vi "Process_Application.vi"(5 "Splash StatusRef":refnum<vi>, 7 "Splash VI Ref":refnum<vi>, 9 "Simulation?":bool, 10 "LaunchState Ev":refnum<user-event>) -> ()   [LabVIEW 2019, in "Application.lvclass"]
doc: "Developed by Kevin Thompson\nkevin@thompsonengineering.net\n\nCopyright 2018\nThompson Engineering, LLC"
uses:
  Application.lvclass
  <vilib>/TELLC/SMQ/Add States to Queue using MultiLine String with vData.vi
  DataTypes/Process - AppData--cluster.ctl
  Common/DataTypes/TD Async CmdMsg EventData--cluster.ctl
  DataTypes/Public Events--cluster.ctl
  DataTypes/Dependency--cluster.ctl
  DataTypes/Settings--cluster.ctl
  Common/Startup/TD LaunchState--enum.ctl
  Common/Startup/TD LaunchData--cluster.ctl
  Common/ErrorHandler/ErrorHandler.lvclass
  Common/DataTypes/TD GetSet ActionSelect--enum.ctl
  Subsystems/Log_Engine/Log_Engine.lvclass
  Subsystems/DAQ_Engine/DAQ_Engine.lvclass
  Subsystems/Main/Main.lvclass
  Subsystems/Config/Config.lvclass
  DataTypes/Read Data--cluster.ctl
panel:
  in  "localData":cluster{"Msg":string, "vData":variant}
  in  "process sync":refnum<notifier>
  out "Application ReadData":T1
  in  "Exit":bool
  in  "Application in":refnum<class "Application.lvclass">
  # "local data monitoring"
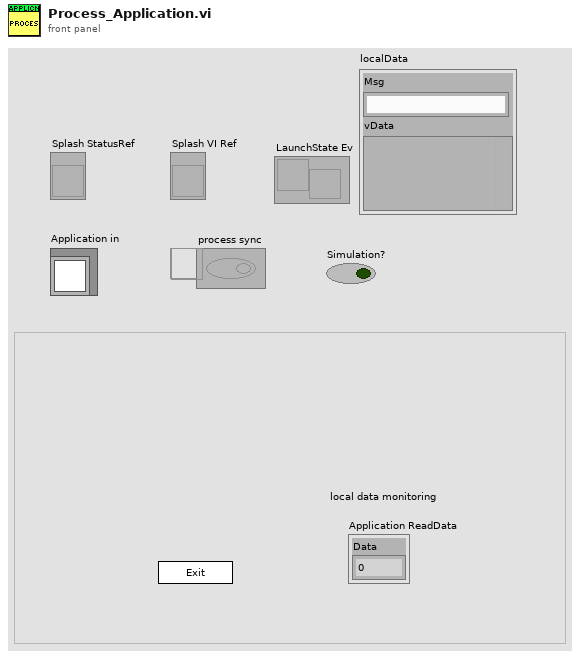
[diagram p1: front panel]
types:
  T1 = typedef "Application.lvclass/Read Data--cluster.ctl" = cluster{"Data":dbl}
  T2 = typedef "TD LaunchData--cluster.ctl" = cluster{"Time Stamp":timestamp, "LaunchState":T3, "Error":errorcluster}
  T3 = typedef "TD LaunchState--enum.ctl" = enum16{"Started", "Stopped"}
  T4 = typedef "Application.lvclass/Process - AppData--cluster.ctl" = cluster{"Core":cluster{"Current VI Reference":refnum<vi>, "Close Panel on Exit?":bool}, "Your Boolean data":bool, "Your string data":string, "SMQ":refnum<queue>, "Initialized?":bool, "Self Reference":refnum<class "Application.lvclass">, "Simulation?":bool, "process sync":refnum<notifier>, "vData":variant, "Public Events":T5, "LaunchState Ev":refnum<user-event>, "RunTimeSystem":bool, "ErrorHandler":refnum<class "ErrorHandler.lvclass">, "Dependency":T6, "StatusMsg Ref":refnum<vi>, "AO IONames":T7, "DO IONames":T8, "UI Labels":T9, "quitting":bool, "DAQEnabled":bool, "Splash StatusRef":refnum<vi>, "Splash VI Ref":refnum<vi>}
  T5 = typedef "Application.lvclass/Public Events--cluster.ctl" = cluster{"Application.AsyncCmd Event":refnum<user-event>, "Application.AsyncMsg Event":refnum<user-event>, "stop process":refnum<user-event>, "Application.ControlStateChg Event":refnum<user-event>, "Application.RadialGraph Event":refnum<user-event>}
  T6 = typedef "Application.lvclass/Dependency--cluster.ctl" = cluster{"Config":refnum<class "Config.lvclass">, "DAQ":refnum<class "DAQ.lvclass">, "Sequencer":refnum<class "Sequencer.lvclass">, "LogEngine":refnum<class "LogEngine.lvclass">, "ErrorHandler":refnum<class "ErrorHandler.lvclass">, "DataQueues":refnum<class "DataQueues.lvclass">, "Motion":refnum<class "Motion.lvclass">, "PID_Ctlr":refnum<class "PID_Ctlr.lvclass">, "Welder":refnum<class "Welder.lvclass">}
  T7 = typedef "AO IONames--cluster.ctl" = cluster{"Weld Current":string, "Turntable Speed":string, "Turntable Jog":string}
  T8 = typedef "DO IONames--cluster.ctl" = cluster{"Arc Enable Relay":string, "AVC Lockout Relay":string, "Turntable Enable Relay":string, "Turntable Jog Switch":string}
  T9 = typedef "UI Controls-Indicators Labels--cluster.ctl" = cluster{"SeqRunning":string, "Process Complete":string, "AVC Lockout":string, "Step Comment":string, "StepCntDn":string, "SeqList":string, "Current SP":string, "VspOffset":string, "WeldCurrentWfmChart":string, "Turntable En (Anlg)":string}
  T10 = typedef "Application.lvclass/Process - AppData--cluster.ctl" = cluster{"Core":cluster{"Current VI Reference":refnum<vi>, "Close Panel on Exit?":bool}, "Your Boolean data":bool, "Your string data":string, "SMQ":refnum<queue>, "Initialized?":bool, "Self Reference":refnum<class "Application.lvclass">, "Simulation?":bool, "process sync":refnum<notifier>, "vData":variant, "Settings":T11, "Dependency":T12, "Public Events":T13, "Splash StatusRef":refnum<vi>, "Splash VI Ref":refnum<vi>, "LaunchState Ev":refnum<user-event>, "ErrorHandler":refnum<class "ErrorHandler.lvclass">, "RunTimeSystem?":bool, "StatusMsg Ref":refnum<vi>}
  T11 = typedef "Application.lvclass/Settings--cluster.ctl" = cluster{"Simulation":bool}
  T12 = typedef "Application.lvclass/Dependency--cluster.ctl" = cluster{"Config":refnum<class "Config.lvclass">, "Main":refnum<class "Main.lvclass">, "ErrorHandler":refnum<class "ErrorHandler.lvclass">, "DAQ_Engine":refnum<class "DAQ_Engine.lvclass">, "Log_Engine":refnum<class "Log_Engine.lvclass">}
  T13 = typedef "Application.lvclass/Public Events--cluster.ctl" = cluster{"Application.AsyncCmd Event":refnum<user-event>, "Application.AsyncMsg Event":refnum<user-event>, "stop process":refnum<user-event>}
  T14 = typedef "TELLC_Temp01.lvclass/Settings--cluster.ctl" = cluster{"Simulation":bool}
  T15 = enum32{"invalid app kind", "Development System", "Run Time System", "Student Edition", "Embedded LabVIEW", "Evaluation", "Custom"}
  T16 = typedef "TD GetSet ActionSelect--enum.ctl" = enum16{"Init", "Get", "Set"}
  T17 = enum32{"Invalid", "Standard", "Closed", "Hidden", "Minimized", "Maximized"}
  T18 = enum32{"Invalid", "Default", "Floating", "Floating/Auto-Hide", "Modal"}
  T19 = typedef "Application.lvclass/AsynCmd_Application--enum.ctl" = enum16{"Application.DoSomething"}
  T20 = typedef "Application.lvclass/AsynMsg_Application--enum.ctl" = enum16{"Application.AppClassReference"}
  T21 = cluster{"Current VI Reference":refnum<vi>, "Close Panel on Exit?":bool}
  T22 = typedef "TD Pathnames--cluster.ctl" = cluster{"RunTimeSys?":bool, "AppFolder":path, "ExecutablePath":path, "ConfigFolder":path, "DataLogFolder":path, "SystemLogFolder":path, "SeqFolder":path, "MainStartupPathname":path, "MainUIPathname":path, "SystemEventsFile":path, "SeqEventsFile":path, "Config SettingsFile":path, "DAQ IOConfigFile":path, "SystemSimulation":bool}
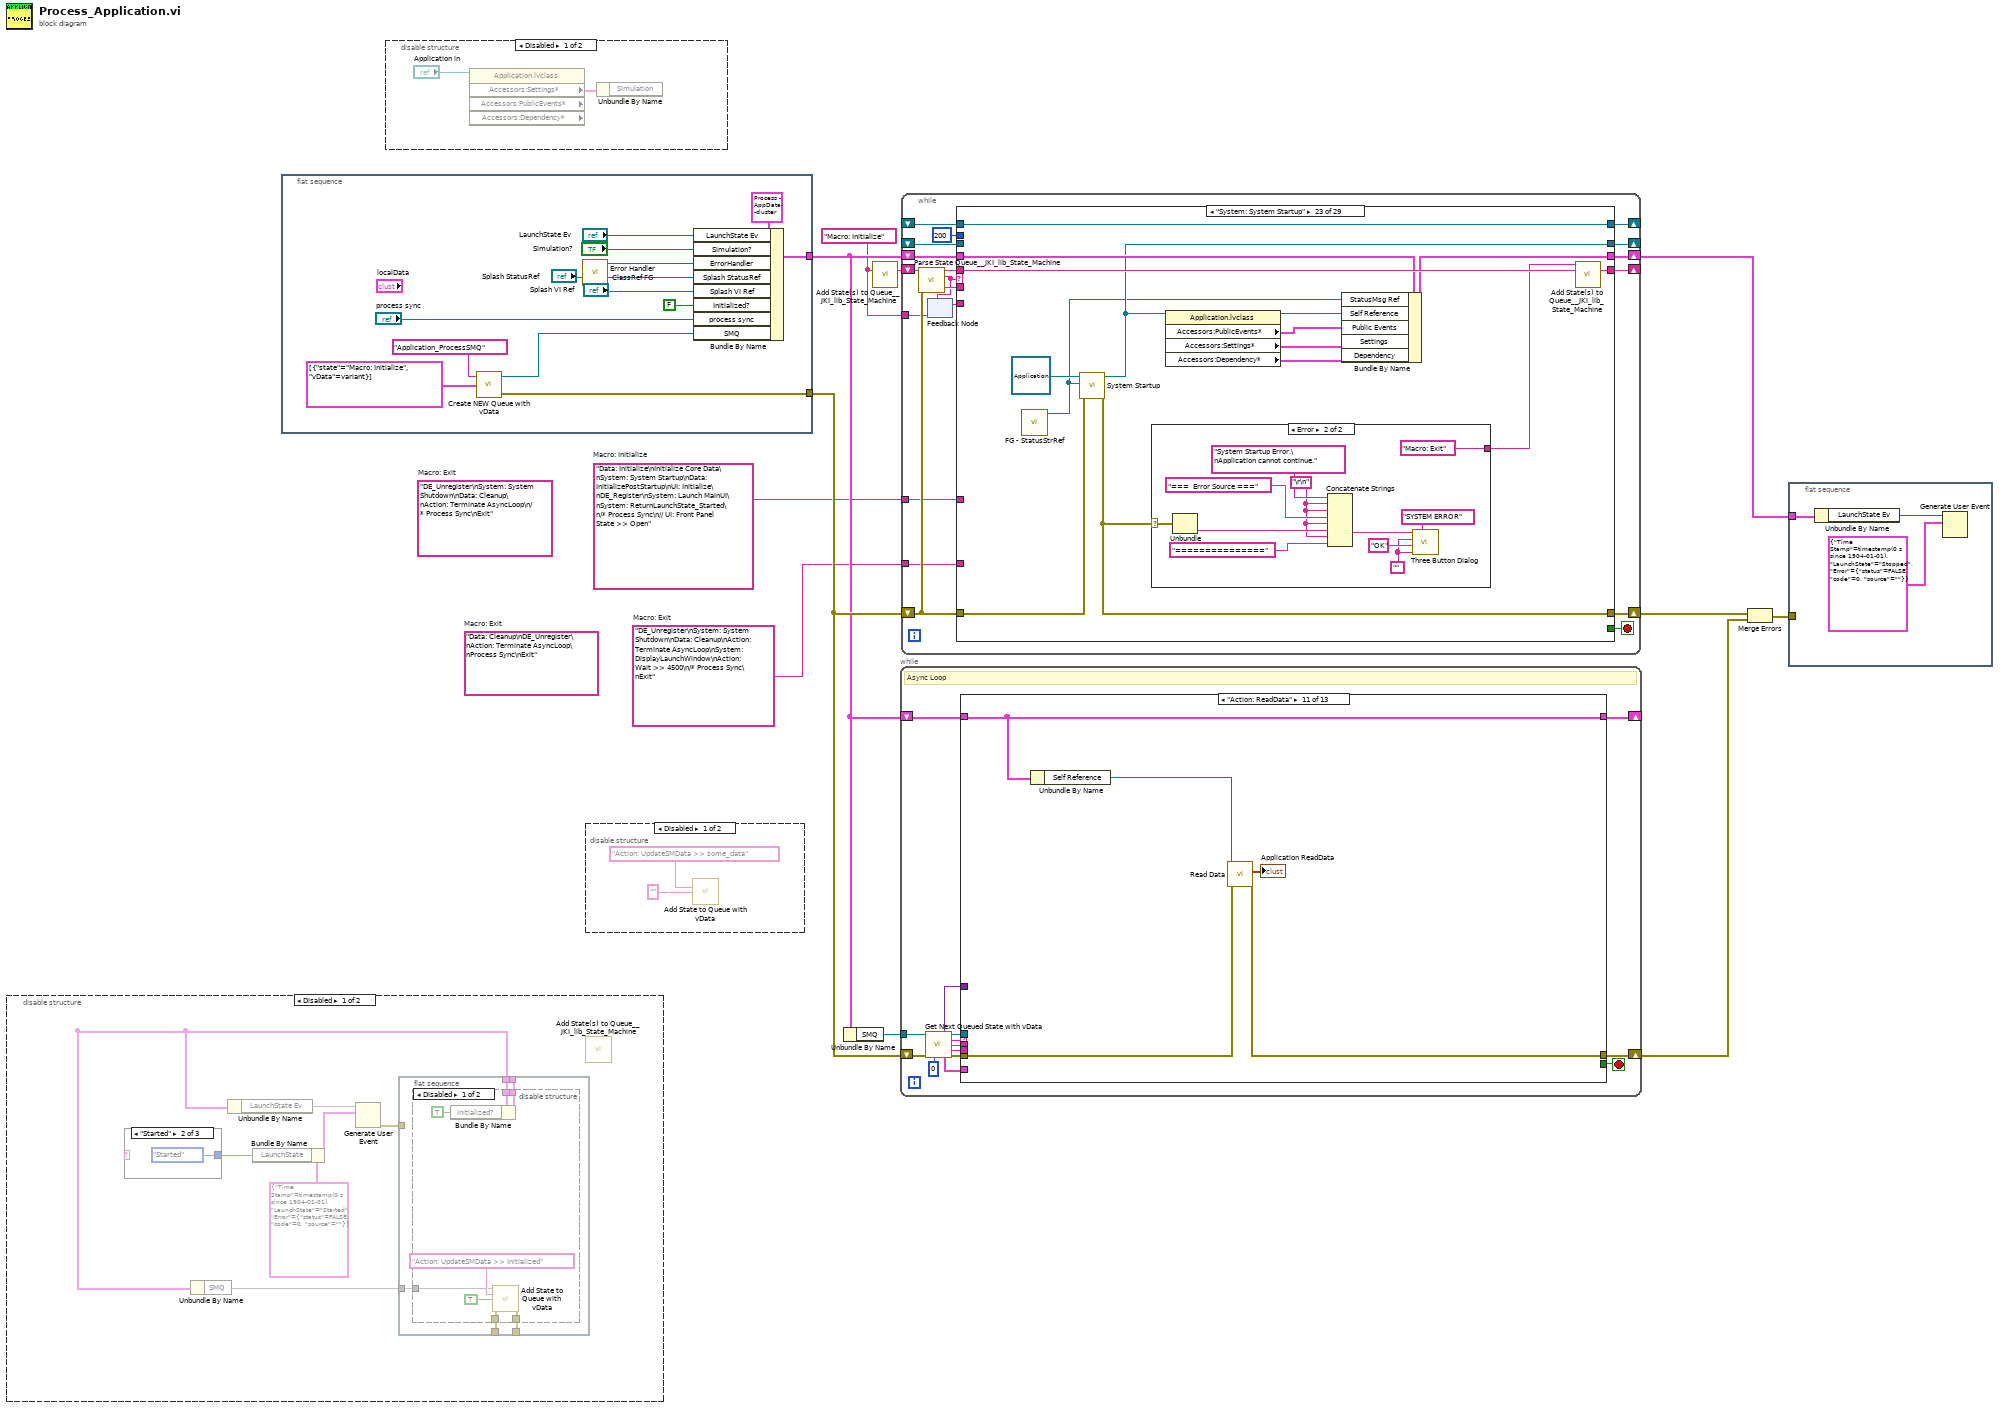
[diagram p0: block diagram]
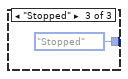
[diagram p4: hidden frame]
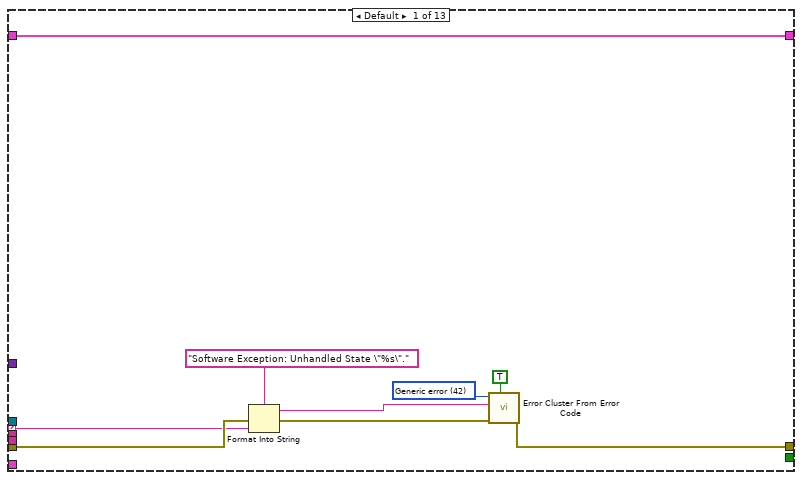
[diagram p8: hidden frame]
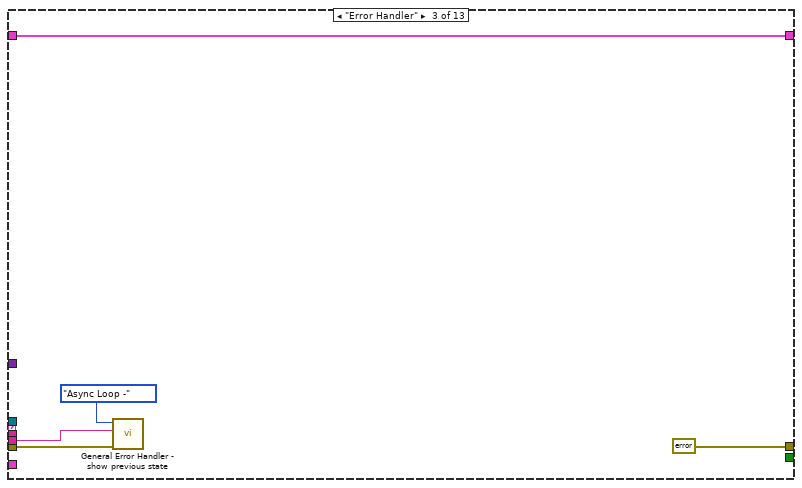
[diagram p10: hidden frame]
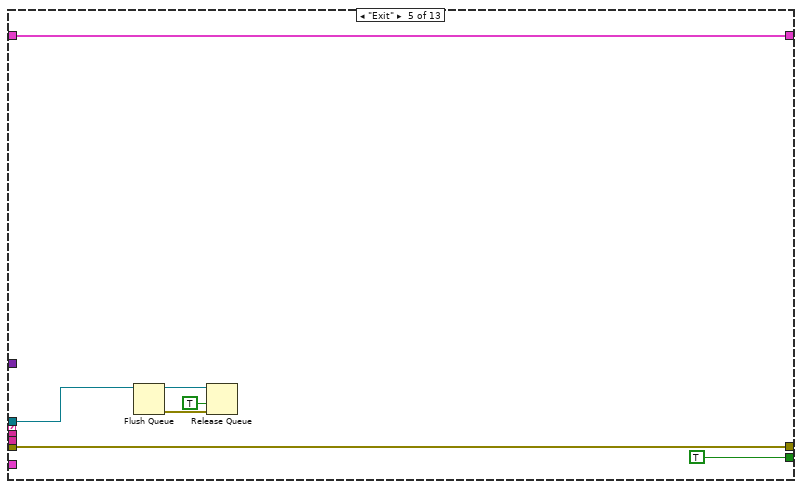
[diagram p12: hidden frame]
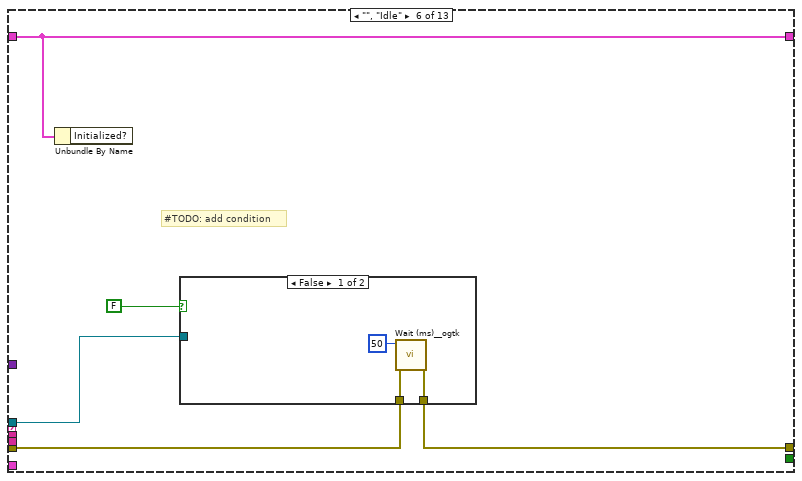
[diagram p13: hidden frame]
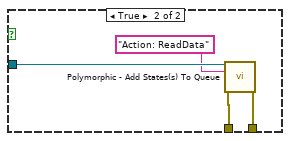
[diagram p14: hidden frame]
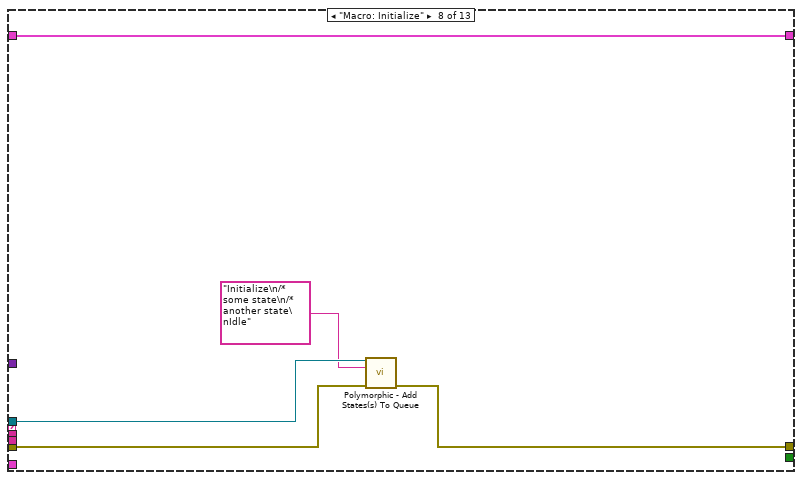
[diagram p16: hidden frame]
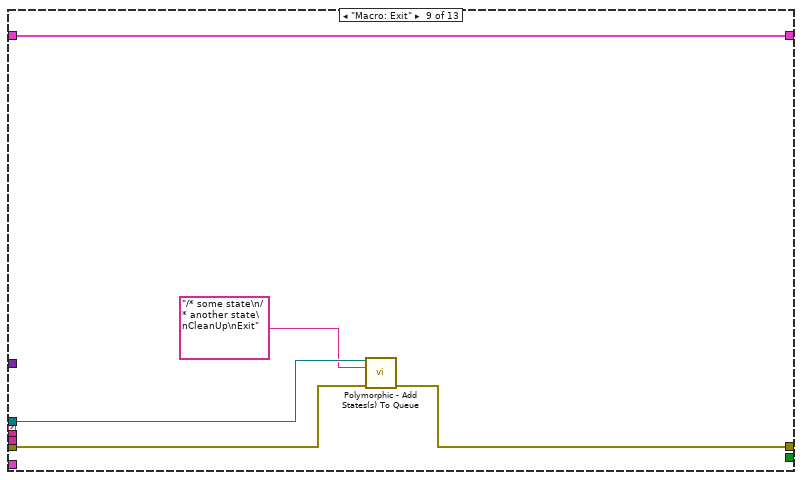
[diagram p17: hidden frame]
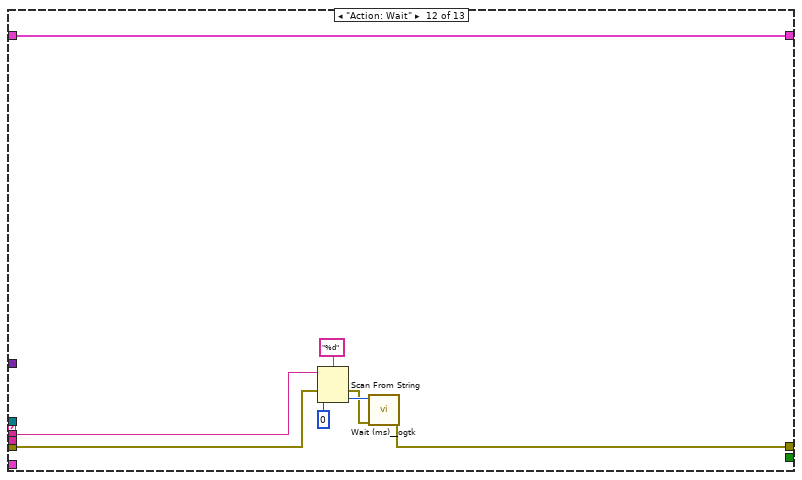
[diagram p19: hidden frame]
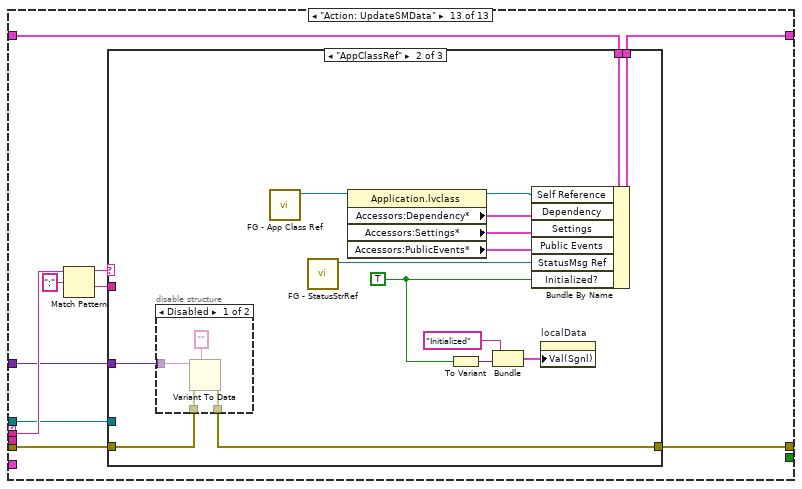
[diagram p20: hidden frame]
diagram:
  w3 = "DE_Unregister\nSystem: System Shutdown\nData: Cleanup\nAction: Terminate AsyncLoop\nSystem: DisplayLaunchWindow\nAction: Wait >> 4500\n/* Process Sync\nExit"  # Macro: Exit
  (unwired) "DE_Unregister\nSystem: System Shutdown\nData: Cleanup\nAction: Terminate AsyncLoop\n/* Process Sync\nExit"  # Macro: Exit
  w4 = "Data: Initialize\nInitialize Core Data\nSystem: System Startup\nData: InitializePostStartup\nUI: Initialize\nDE_Register\nSystem: Launch MainUI\nSystem: ReturnLaunchState_Started\n/* Process Sync\n// UI: Front Panel State >> Open"  # Macro: Initialize
  (unwired) "Data: Cleanup\nDE_Unregister\nAction: Terminate AsyncLoop\nProcess Sync\nExit"  # Macro: Exit
  w5 = "Macro: Initialize"
  n1 = disable-structure shown="Disabled" {
    frame Disabled {
      n2 = case shown="\"Started\"" w19 {
        tunnel: [_ TD_LaunchState--enum."Started" ("LaunchState") TD_LaunchState--enum."Stopped" ("LaunchState")] -> w22
        frame Default {
        }
        frame "Started" {
        }
        frame "Stopped" {
        }
      }
      n3 = Unbundle By Name() -> (w13:T4, "LaunchState Ev"=w20)
      n4 = Unbundle By Name(w13) -> ("SMQ"=w12)
      n5 = Bundle By Name(cluster=T2 {"Time Stamp"=timestamp(0 s since 1904-01-01), "LaunchState"=enum."Started", "Error"={"status"=FALSE, "code"=0, "source"=""}} ("LaunchData"), "LaunchState"=w22) -> (w21:T2)
      n6 = Generate User Event(user event=w20, event data cluster=w21) -> (error out=w16:errorcluster)  [unwired: 2 in, 1 out]
      n7 = flat-sequence {
        tunnel: w13 -> [w28]
        tunnel: [w27] -> w17
        tunnel: w16 -> [_]
        tunnel: [w26] -> w15
        tunnel: [w25] -> w14
        tunnel: w12 -> [w24]
        frame #0 {
          n8 = disable-structure shown="Disabled" {
            disable-tunnel: w28 -> [w36 w38]
            disable-tunnel: [w35 w38] -> w27
            disable-tunnel: w26 -> [w31 w37]
            disable-tunnel: [w30 w37] -> w25
            disable-tunnel: w24 -> [w29 _]
            frame Disabled {
              n9 = Bundle By Name(cluster=w36, "Initialized?"=TRUE) -> (w35:cluster{})
              n10 = call <vilib>:"Add State to Queue with vData.vi"("queue in"=w29, "state in"="Action: UpdateSMData >> Initialized", "vData (\"\")"=TRUE, "error in"=w31) -> ("error out"=w30:errorcluster)  [unwired: 8 in, 3 out]
            }
            frame Enabled {
            }
          }
        }
      }
      n11 = call <vilib>:"Add State(s) to Queue__JKI_lib_State_Machine.vi"() -> ("State(s) in (\"\")"=w23:string)  [unwired: 14 in, 1 out]
    }
    frame Enabled {
    }
  }
  n12 = flat-sequence {
    tunnel: [w53] -> w8
    tunnel: [w50] -> w10
    frame #0 {
      n13 = call <vilib>:"Create NEW Queue with vData.vi"("Initial States"=cluster{"state":string, "vData":variant}[] [{"state"="Macro: Initialize", "vData"=variant}], "Name (SMQ)"="Application_ProcessSMQ") -> ("error out"=w50:errorcluster, "queue out"=w52:refnum<queue>)  [unwired: 2 in]
      n14 = call "Error Handler ClassRef FG.vi"() -> ("ErrorHandler out"=w43:refnum<class "ErrorHandler.lvclass">)  [unwired: 10 in, 1 out]
      n15 = Bundle By Name(cluster=T10 {"Core"={"Current VI Reference"=refnum, "Close Panel on Exit?"=FALSE}, "Your Boolean data"=FALSE, "Your string data"="", "SMQ"=refnum, "Initialized?"=FALSE, "Self Reference"=refnum, "Simulation?"=FALSE, "process sync"=refnum, "vData"=variant, "Settings"={"Simulation"=FALSE}, "Dependency"={"Config"=refnum, "Main"=refnum, "ErrorHandler"=refnum, "DAQ_Engine"=refnum, "Log_Engine"=refnum}, "Public Events"={"Application.AsyncCmd Event"=refnum, "Application.AsyncMsg Event"=refnum, "stop process"=refnum}, "Splash StatusRef"=refnum, "Splash VI Ref"=refnum, "LaunchState Ev"=refnum, "ErrorHandler"=refnum, "RunTimeSystem?"=FALSE, "StatusMsg Ref"=refnum} ("SM2 AppData"), "LaunchState Ev"="LaunchState Ev", "Simulation?"="Simulation?", "ErrorHandler"=w43, "Splash StatusRef"="Splash StatusRef", "Splash VI Ref"="Splash VI Ref", "Initialized?"=FALSE, "process sync"="process sync", "SMQ"=w52) -> (w53:T10)
    }
  }
  n16 = disable-structure shown="Disabled" {
    frame Disabled {
      n17 = property class="Application.lvclass" props=["Accessors:Settings*", "Accessors:PublicEvents*", "Accessors:Dependency*"](reference="Application in") -> ("Accessors:Settings*"=w55:T14)  [unwired: 1 in, 4 out]
      n18 = Unbundle By Name(w55) -> ()  [unwired: 1 out]
    }
    frame Enabled {
    }
  }
  n19 = disable-structure shown="Disabled" {
    frame Disabled {
      n20 = call <vilib>:"Add State to Queue with vData.vi"("state in"="Action: UpdateSMData >> some_data", "vData (\"\")"="") -> ()  [unwired: 10 in, 4 out]
    }
    frame Enabled {
    }
  }
  n21 = Unbundle By Name(w8) -> ("SMQ"=w9:refnum<queue>)
  n22 = call <vilib>:"Add State(s) to Queue__JKI_lib_State_Machine.vi"("State(s) in (\"\")"=w5) -> ("States Out"=w11:string)  [unwired: 14 in]
  n23 = while {
    shift-right: [w68] -> w6
    shift-left: w10 -> [w70]
    tunnel: w9 -> [w66]
    shift-right: [w64] -> _
    shift-left: w8 -> [w65]
    stop <- w59 stop-if-true
    # "Async Loop"
    n24 = call <vilib>:"Get Next Queued State with vData.vi"("queue in"=w66, "error in (no error)"=w70, "timeout (100)"=0) -> ("vData out"=w63:variant, "queue out"=w67:refnum<queue>, "Next State"=w71:string, "queued msg"=w61:string, "Prev State"=w60:string, "RemainingElements"=w58:cluster{"state":string, "vData":variant}[], "error out"=w69:errorcluster)  [unwired: 6 in]
    n25 = case shown="\"Action: ReadData\"" w71 {
      tunnel: w67 -> [_ _ _ _ w90 w98 _ w114 w119 _ _ _ w141]
      tunnel: w61 -> [_ _ _ _ _ _ _ _ _ _ _ w130 w143]
      selector: w71 -> [w72 _ _ _ _ _ _ _ _ _ _ _ _]
      tunnel: w69 -> [w74 w82 w84 w89 w96 w101 w110 w113 w118 w122 w125 w129 w138]
      tunnel: [w73 w82 errorcluster {"status"=FALSE, "code"=0, "source"=""} ("error constant") w89 w96 w100 w110 w112 w117 w122 w124 w132 w137] -> w68
      tunnel: w65 -> [w80 w81 w87 w88 w95 w97 w109 w115 w120 w121 w127 w135 w140]
      tunnel: [w80 w81 w87 w88 w95 w97 w109 w115 w120 w121 w127 w135 w139] -> w64
      tunnel: w63 -> [_ _ _ _ _ _ _ _ _ _ _ _ w142]
      tunnel: w60 -> [_ _ w83 _ _ _ _ _ _ _ _ _ _]
      tunnel: [_ _ _ _ TRUE _ _ _ _ _ _ _ _] -> w59
      tunnel: w58 -> [_ _ _ _ _ _ _ _ _ _ _ _ _]
      frame Default {
        w76 = 42 items=["No error", "Argument error", "Memory is full", "Out of zone", "End of file", "File already open", "Generic file I/O error", "File not found", "File permission error", "Disk is full", "Duplicate path", "Too many files open", "System feature not enabled", "Resource file not found", "Cannot add resource", "Resource not found", "Image not found", "Image memory error", "Pen does not exist", "Config type invalid", "Config token not found", "Config parse error", "Config memory error", "Bad external code format", "Bad external code offset", "External code not present", "Null window", "Destroy window error", "Null menu", "Print aborted", "Bad print record", "Print driver error", "Windows error during printing", "Memory error during printing", "Print dialog error", "Generic print error", "Invalid device refnum", "Device not found", "Device parameter error", "Device unit error", "Cannot open device", "Device call aborted", "Generic error", "Cancelled by user", "Object ID too low", "Object ID too high", "Object not in heap", "Unknown heap", "Unknown object (invalid DefProc)", "Unknown object (DefProc not in table)", "Message out of range", "Invalid (null) method", "Unknown message", "Manager call not supported", "Bad address", "Network operation in progress", "Network operation timed out", "Connection is busy", "Network attribute not supported", "Network error", "Address in use", "System out of memory", "Connection aborted", "Connection refused", "Not connected", "Already connected", "Connection closed", "Initialization error (interapplication manager)", "Bad occurrence", "Wait on unbound occurrence handler", "Occurrence queue overflow", "Datalog type conflict", "Unused", "Unrecognized type (interapplication manager)", "Memory corrupt", "Failed to make temporary DLL", "Old CIN version", "Drag socket not found", "Failed to load drop-object", "Failed to register OLE object", "Failed to release OLE object", "Format specifier type mismatch", "Unknown format specifier", "Too few format specifiers", "Too many format specifiers", "Scan failed", "Newer CIN version", "Error converting to variant", "Runtime menu error", "Password tampered", "Variant attribute not found", "Incompatible variant data type", "Event data is not available", "Event Store is not present", "Occurrence is not found", "Event Queue is not created", "Event info is not available", "Refnum passed is NULL", "Error retrieving Class GUID", "Error retrieving CoClass GUID", "Error retrieving TypeLib GUID.", "Bad built application magic bytes.", "Specific driver is different from the specific driver associated with the Logical Name.", "There is no session opened to the class driver.", "Max Error", "MAX - Error with config objects", "MAX - Error loading configuration", "MAX - Group not supported"]
        n26 = Format Into String(format string="Software Exception: Unhandled State \"%s\"." ("message"), error in=w74, w72) -> (resulting string=w77:string, error out=w78:errorcluster)  [unwired: 1 in]
        n27 = call <vilib>:"Error Cluster From Error Code.vi"("show call chain? (False)"=TRUE, "error in (no error)"=w78, "error message (\"\")"=w77, "error code (0)"=w76) -> ("error out"=w73:errorcluster)  [unwired: 5 in]
      }
      frame "Initialize" {
      }
      frame "Error Handler" {
        n28 = call "General Error Handler - show previous state.vi"("error in (no error)"=w84, "Previous State"=w83, "Loop Select"=enum16{"Event Loop -", "Async Loop -"}."Async Loop -") -> ()  [unwired: 7 in, 2 out]
      }
      frame "CleanUp" {
      }
      frame "Exit" {
        n29 = Flush Queue(queue=w90) -> (queue out=w93:refnum<queue>, error out=w92:errorcluster)  [unwired: 1 in, 1 out]
        n30 = Release Queue(queue=w93, force destroy? (F)=TRUE, error in (no error)=w92) -> ()  [unwired: 3 out]
      }
      frame "", "Idle" {
        # "#TODO: add condition"
        n31 = Unbundle By Name(w97) -> ()  [unwired: 1 out]
        n32 = case shown="False" FALSE {
          tunnel: w101 -> [w104 w108]
          tunnel: [w103 w107] -> w100
          tunnel: w98 -> [_ w106]
          frame False {
            n33 = call <userlib>:"Wait (ms)__ogtk.vi"("error in (no error)"=w104, "milliseconds to wait"=u32 50) -> ("error out"=w103:errorcluster)  [unwired: 8 in, 1 out]
          }
          frame True {
            n34 = call-poly <vilib>:"Polymorphic - Add States(s) To Queue.vi"("queue in"=w106, "state in"="Action: ReadData", "error in"=w108) -> ("error out"=w107:errorcluster)  [unwired: 9 in, 3 out]
          }
        }
      }
      frame "------ Macro ------" {
      }
      frame "Macro: Initialize" {
        n35 = call-poly <vilib>:"Polymorphic - Add States(s) To Queue.vi"("queue in"=w114, "states in"="Initialize\n/* some state\n/* another state\nIdle", "error in"=w113) -> ("error out"=w112:errorcluster)  [unwired: 10 in, 2 out]
      }
      frame "Macro: Exit" {
        n36 = call-poly <vilib>:"Polymorphic - Add States(s) To Queue.vi"("queue in"=w119, "states in"="/* some state\n/* another state\nCleanUp\nExit", "error in"=w118) -> ("error out"=w117:errorcluster)  [unwired: 10 in, 2 out]
      }
      frame "------ Action ------" {
      }
      frame "Action: ReadData" {
        n37 = Unbundle By Name(w127) -> ("Self Reference"=w126:refnum<class "Application.lvclass">)
        n38 = call "Read Data.vi"("error in (no error)"=w125, "Application in"=w126) -> ("error out"=w124:errorcluster, "Application ReadData"=→"Application ReadData":T1)  [unwired: 7 in, 1 out]
      }
      frame "Action: Wait" {
        n39 = Scan From String(format string="%d", input string=w130, error in=w129, default 1=u32 0) -> (error out=w128:errorcluster, output 1=w134:u32)  [unwired: 1 in, 2 out]
        n40 = call <userlib>:"Wait (ms)__ogtk.vi"("error in (no error)"=w128, "milliseconds to wait"=w134) -> ("error out"=w132:errorcluster)  [unwired: 8 in, 1 out]
      }
      frame "Action: UpdateSMData" {
        n41 = Match Pattern(string=w143, regular expression=":") -> (before substring=w145:string, after substring=w136:string)  [unwired: 1 in, 2 out]
        n42 = case shown="\"AppClassRef\"" w145 {
          tunnel: w142 -> [_ w162 w174]
          tunnel: w141 -> [_ _ _]
          tunnel: w140 -> [w146 w159 w171]
          tunnel: [w146 w158 w170] -> w139
          tunnel: w138 -> [w147 w161 w173]
          tunnel: [w147 w160 w172] -> w137
          tunnel: w136 -> [_ _ _]
          frame Default {
            # "#NOTE:\noptionally add error here."
          }
          frame "AppClassRef" {
            w152 = TRUE
            n43 = disable-structure shown="Disabled" {
              disable-tunnel: w162 -> [w166 _]
              disable-tunnel: w161 -> [w164 w167]
              disable-tunnel: [w163 w167] -> w160
              frame Disabled {
                n44 = Variant To Data(error in=w164, type="", Variant=w166) -> (error out=w163:errorcluster)  [unwired: 1 out]
              }
              frame Enabled {
              }
            }
            n45 = call "FG - App Class Ref.vi"() -> ("Application out"=w156:refnum<class "Application.lvclass">)  [unwired: 9 in, 1 out]
            n46 = call "FG - StatusStrRef.vi"() -> ("StatusStr Ref out"=w157:refnum<vi>)  [unwired: 9 in, 1 out]
            n47 = property class="Application.lvclass"(reference=w156) -> (reference out=w151:refnum<class "Application.lvclass">, "Accessors:Dependency*"=w150:T12, "Accessors:Settings*"=w149:T11, "Accessors:PublicEvents*"=w148:T13)  [unwired: 1 in, 1 out]
            n48 = To Variant(anything=w152) -> (Variant=w154:variant)
            n49 = Bundle("Initialized", "Variant"=w154) -> (w153:cluster{string, "Variant":variant})  [unwired: 1 in]
            n50 = Bundle By Name(cluster=w159, "Self Reference"=w151, "Dependency"=w150, "Settings"=w149, "Public Events"=w148, "StatusMsg Ref"=w157, "Initialized?"=w152) -> (w158:T10)
            n51 = property on="localData" class="Clust (strict)"("Val(Sgnl)"=w153) -> ()  [unwired: 2 in, 2 out]
          }
          frame "Dependency" {
            n52 = Variant To Data(error in=w173, type=T12 {"Config"=refnum, "Main"=refnum, "ErrorHandler"=refnum, "DAQ_Engine"=refnum, "Log_Engine"=refnum} ("Dependency"), Variant=w174) -> (data=w168:T12, error out=w172:errorcluster)
            n53 = Bundle By Name(cluster=w171, "Dependency"=w168) -> (w170:T10)
          }
        }
      }
    }
  }
  n54 = while {
    shift-right: [w187] -> w1
    shift-left: w8 -> [w186]
    shift-right: [w190] -> w7
    shift-left: w10 -> [w185]
    shift-right: [w189] -> _
    shift-left: w11 -> [w191]
    shift-right: [w184] -> _
    shift-left: _ -> [w183]
    tunnel: w4 -> [w181]
    tunnel: w3 -> [w180]
    tunnel: w5 -> [w179]
    shift-right: [w176] -> _
    shift-left: _ -> [w175]
    stop <- w188 stop-if-true
    n55 = call <vilib>:"Parse State Queue__JKI_lib_State_Machine.vi"("State Queue"=w191, "Error In (no error)"=w185) -> ("Remaining States"=w193:string, "Current State"=w178:string, "Arguments"=w192:string)  [unwired: 11 in]
    n56 = feedback #1(w179) -> (w177:string)
    n57 = feedback-in #1(w178) -> ()
    n58 = case shown="\"System: System Startup\"" w178 {
      selector: w178 -> [w196 _ _ _ _ _ _ _ _ _ _ _ _ _ _ _ _ _ _ _ _ _ _ _ _ _ _ _ _]
      tunnel: w193 -> [w200 w216 w225 w234 w349 w361 w375 w381 w386 w392 w404 w414 w423 w429 w438 w448 w461 w489 w496 w508 w514 w538 w553 w585 w590 w625 w631 w643 w653]
      tunnel: w192 -> [_ _ _ _ _ _ _ _ _ _ _ _ _ _ _ w443 w455 _ _ _ _ _ _ _ w589 _ _ w633 _]
      tunnel: w186 -> [w198 w213 w217 w232 w346 w355 w372 w378 w385 w389 w394 w406 w418 w426 w433 w446 w457 w486 w493 w505 w511 w530 w548 w571 w591 w623 w628 w641 w650]
      tunnel: [w202 errorcluster {"status"=FALSE, "code"=0, "source"=""} ("error out") w223 w231 w347 w358 w368 w379 w383 w390 w397 w412 w419 w427 w434 w444 w458 w487 w494 w506 w512 w515 w547 w569 w588 w620 w629 w634 w645] -> w190
      tunnel: w185 -> [w201 w208 w223 w230 w347 w358 w369 _ w383 w390 w396 w412 w420 w427 w435 w445 w459 w487 w494 w506 w512 w529 w546 w569 w587 w619 w629 w635 w646]
      tunnel: [w199 w215 w224 w233 w348 w360 w374 w381 w386 w391 w403 w413 w422 w428 w437 w447 w460 w488 w495 w507 w513 w537 w552 w584 w592 w624 w630 w642 w652] -> w189
      tunnel: [_ _ TRUE _ _ _ _ _ _ _ _ _ _ _ _ _ _ _ _ _ _ _ _ _ _ _ _ _ _] -> w188
      tunnel: [w198 w213 w217 w229 w346 w359 w372 w378 w385 w389 w395 w408 w418 w426 w433 w446 w457 w486 w493 w505 w511 w530 w549 w571 w593 w623 w628 w641 w650] -> w187
      tunnel: [w195 w211 w221 w227 w345 w352 w373 w380 w384 w388 w402 w407 w417 w425 w436 w442 w454 w485 w492 w499 w510 w536 w551 w583 w601 w622 w627 w640 w651] -> w184
      tunnel: w183 -> [w195 w211 w221 w227 w345 w352 w373 _ w384 w388 w402 w407 w417 w425 w436 w442 w454 w485 w492 w499 w510 w536 w551 w583 w601 w622 w627 w640 w651]
      tunnel: 200 ("Timeout") -> [_ _ _ w228 _ _ _ _ _ _ _ _ _ _ _ _ _ _ _ _ _ _ _ _ _ _ _ _ _]
      tunnel: w181 -> [_ _ _ _ _ _ _ _ _ _ _ _ _ _ _ _ _ _ w491 _ _ _ _ _ _ _ _ _ _]
      tunnel: w180 -> [_ _ _ _ _ _ _ _ _ _ _ _ _ _ _ _ _ _ _ w498 _ _ _ _ _ _ _ _ _]
      tunnel: w177 -> [_ w207 _ _ _ _ _ _ _ _ _ _ _ _ _ _ _ _ _ _ _ _ _ _ _ _ _ _ _]
      tunnel: [w194 w210 w220 w226 w344 w350 w367 w376 w382 w387 w399 w405 w416 w424 w430 w441 w453 w484 w490 w497 w509 w535 w545 w567 w600 w621 w626 w632 w644] -> w176
      tunnel: w175 -> [w194 w210 w220 w226 w344 w350 w367 w376 w382 w387 w398 w405 w416 w424 w430 w441 w453 w484 w490 w497 w509 w535 _ w567 w600 w621 w626 w632 w644]
      frame Default {
        w205 = 42 items=["No error", "Argument error", "Memory is full", "Out of zone", "End of file", "File already open", "Generic file I/O error", "File not found", "File permission error", "Disk is full", "Duplicate path", "Too many files open", "System feature not enabled", "Resource file not found", "Cannot add resource", "Resource not found", "Image not found", "Image memory error", "Pen does not exist", "Config type invalid", "Config token not found", "Config parse error", "Config memory error", "Bad external code format", "Bad external code offset", "External code not present", "Null window", "Destroy window error", "Null menu", "Print aborted", "Bad print record", "Print driver error", "Windows error during printing", "Memory error during printing", "Print dialog error", "Generic print error", "Invalid device refnum", "Device not found", "Device parameter error", "Device unit error", "Cannot open device", "Device call aborted", "Generic error", "Cancelled by user", "Object ID too low", "Object ID too high", "Object not in heap", "Unknown heap", "Unknown object (invalid DefProc)", "Unknown object (DefProc not in table)", "Message out of range", "Invalid (null) method", "Unknown message", "Manager call not supported", "Bad address", "Network operation in progress", "Network operation timed out", "Connection is busy", "Network attribute not supported", "Network error", "Address in use", "System out of memory", "Connection aborted", "Connection refused", "Not connected", "Already connected", "Connection closed", "Initialization error (interapplication manager)", "Bad occurrence", "Wait on unbound occurrence handler", "Occurrence queue overflow", "Datalog type conflict", "Unused", "Unrecognized type (interapplication manager)", "Memory corrupt", "Failed to make temporary DLL", "Old CIN version", "Drag socket not found", "Failed to load drop-object", "Failed to register OLE object", "Failed to release OLE object", "Format specifier type mismatch", "Unknown format specifier", "Too few format specifiers", "Too many format specifiers", "Scan failed", "Newer CIN version", "Error converting to variant", "Runtime menu error", "Password tampered", "Variant attribute not found", "Incompatible variant data type", "Event data is not available", "Event Store is not present", "Occurrence is not found", "Event Queue is not created", "Event info is not available", "Refnum passed is NULL", "Error retrieving Class GUID", "Error retrieving CoClass GUID", "Error retrieving TypeLib GUID.", "Bad built application magic bytes.", "Specific driver is different from the specific driver associated with the Logical Name.", "There is no session opened to the class driver.", "Max Error", "MAX - Error with config objects", "MAX - Error loading configuration", "MAX - Group not supported"]
        # "Current State"
        n59 = Format Into String(format string="Software Exception: Unhandled State \"%s\"." ("message"), error in=w201, w196) -> (resulting string=w204:string, error out=w203:errorcluster)  [unwired: 1 in]
        n60 = call <vilib>:"Error Cluster From Error Code.vi"("show call chain? (False)"=TRUE, "error in (no error)"=w203, "error message (\"\")"=w204, "error code (0)"=w205) -> ("error out"=w202:errorcluster)  [unwired: 5 in]
        n61 = call <vilib>:"Add State(s) to Queue__JKI_lib_State_Machine.vi"("State(s) in (\"\")"=w200) -> ("States Out"=w199:string)  [unwired: 14 in]
      }
      frame "Error Handler" {
        n62 = call "General Error Handler - show previous state.vi"("error in (no error)"=w208, "Previous State"=w207, "Loop Select"=enum16{"Event Loop -", "Async Loop -"}."Event Loop -") -> ()  [unwired: 7 in, 2 out]
        n63 = call <vilib>:"Add State(s) to Queue__JKI_lib_State_Machine.vi"("State(s) in Front (\"\")"="/* Post Error States", "State(s) in (\"\")"=w216) -> ("States Out"=w215:string)  [unwired: 13 in]
      }
      frame "Exit" {
        n64 = Unbundle By Name(w217) -> ("StatusMsg Ref"=w218:refnum<vi>)
        n65 = call <vilib>:"format status message v2.vi"("status msg"="System shutdown complete", "Str Refnum"=w218) -> ()  [unwired: 5 in, 5 out]
        n66 = call <vilib>:"Add State(s) to Queue__JKI_lib_State_Machine.vi"("State(s) in (\"\")"=w225) -> ("States Out"=w224:string)  [unwired: 14 in]
      }
      frame "", "Event Structure", "Idle" {
        n67 = event shown="[7] <Public Events.Application.AsyncMsg Event>: User Event" {
          selector: w227 -> [_ _ _ _ _ _ _ _]
          dyn-events: _ -> [_ _ _ _ _ _ _ _]
          timeout: w228 -> [_ _ _ _ _ _ _ _]
          tunnel: w234 -> [w238 w243 w249 w252 w264 w276 w293 w323]
          tunnel: [w237 w242 w248 w251 w264 w275 w292 w322] -> w233
          tunnel: w232 -> [w235 w240 w246 w254 w257 w279 w282 w312]
          tunnel: [w236 w241 w247 w255 w259 w280 w290 w320] -> w231
          tunnel: w230 -> [w236 w241 w247 w255 w260 w280 w289 w319]
          tunnel: [w235 w240 w246 w254 w258 w278 w284 w314] -> w229
          event Timeout {
            n68 = event-data() -> ()  [unwired: 1 in, 1 out]
            n69 = call <vilib>:"Add State(s) to Queue__JKI_lib_State_Machine.vi"("State(s) in (\"\")"=w238) -> ("States Out"=w237:string)  [unwired: 14 in]
          }
          event "Exit": Value Change {
            n70 = event-data() -> ()  [unwired: 1 in, 1 out]
            n71 = call <vilib>:"Add State(s) to Queue__JKI_lib_State_Machine.vi"("State(s) in Front (\"\")"="Macro: Exit", "State(s) in (\"\")"=w243) -> ("States Out"=w242:string)  [unwired: 13 in]
          }
          event Panel Close? {
            n72 = event-data() -> ()  [unwired: 1 in, 1 out]
            n73 = call <vilib>:"Add State(s) to Queue__JKI_lib_State_Machine.vi"("State(s) in Front (\"\")"="Macro: Exit", "State(s) in (\"\")"=w249) -> ("States Out"=w248:string)  [unwired: 13 in]
            n74 = event-data("Discard?"=TRUE) -> ()  [unwired: 1 in, 1 out]
          }
          event Menu Selection (User) {
            n75 = event-data() -> ("ItemTag"=w253:string)  [unwired: 1 in, 2 out]
            n76 = case shown="\"False\", Default" w253 {
              tunnel: [""] -> w250
              frame "False", Default {
              }
            }
            n77 = call <vilib>:"Add State(s) to Queue__JKI_lib_State_Machine.vi"("State(s) in Front (\"\")"=w250, "State(s) in (\"\")"=w252) -> ("States Out"=w251:string)  [unwired: 13 in]
          }
          event "localData": Value Change {
            n78 = event-data() -> ("NewVal"=w263:cluster{"Msg":string, "vData":variant})  [unwired: 1 in]
            n79 = Unbundle(w263) -> ("Msg"=w262:string, "vData"=w261:variant)
            n80 = case shown="\"Initialized\"" w262 {
              tunnel: w261 -> [_ w273]
              tunnel: w260 -> [w266 w272]
              tunnel: [w266 w271] -> w259
              tunnel: w257 -> [w265 w270]
              tunnel: [w265 w269] -> w258
              frame "False", Default {
              }
              frame "Initialized" {
                n81 = Variant To Data(error in=w272, type=FALSE, Variant=w273) -> (data=w267:bool, error out=w271:errorcluster)
                n82 = Bundle By Name(cluster=w270, "Initialized?"=w267) -> (w269:T10)
              }
            }
          }
          event User Event {
            n83 = event-data() -> ("notifier out"=w277:refnum<notifier>)  [unwired: 1 in]
            n84 = Bundle By Name(cluster=w279, "process sync"=w277) -> (w278:T10)
            n85 = call <vilib>:"Add State(s) to Queue__JKI_lib_State_Machine.vi"("State(s) in Front (\"\")"="Macro: Exit", "State(s) in (\"\")"=w276) -> ("States Out"=w275:string)  [unwired: 13 in]
          }
          event User Event {
            n86 = event-data() -> ("CmdMsg"=w287:string, "vData"=w291:variant)  [unwired: 1 in, 1 out]
            n87 = Unbundle By Name(w282) -> ("Self Reference"=w283:refnum<class "Application.lvclass">, "SMQ"=w281:refnum<queue>)
            n88 = call "get async cmd.vi"("error in (no error)"=w289, "Cmd String in"=w287) -> ("error out"=w288:errorcluster, "AsyncCmd"=w286:T19)  [unwired: 8 in]
            n89 = case shown="\"Application.DoSomething\"" w286 {
              tunnel: w291 -> [_ w306]
              tunnel: w288 -> [w299 w305]
              tunnel: [w298 w304] -> w290
              tunnel: [_ ""] -> w285
              tunnel: w282 -> [w294 w302]
              tunnel: [w294 w301] -> w284
              tunnel: w283 -> [_ _]
              tunnel: w282 -> [_ _]
              tunnel: w281 -> [_ _]
              frame Default {
                n90 = call <vilib>:"Build Error Cluster_ModKT .vi"("Prepend String (\"\")"="Invalid Async Cmd" ("Prepend String (\"\")"), "code"=42, "error? (F)"=TRUE, "error in (no error)"=w299) -> ("error out"=w298:errorcluster)  [unwired: 3 in, 1 out]
              }
              frame "Application.DoSomething" {
                n91 = disable-structure shown="Disabled" {
                  disable-tunnel: w306 -> [w309 _]
                  disable-tunnel: w305 -> [w308 w310]
                  disable-tunnel: [w307 w310] -> w304
                  frame Disabled {
                    n92 = Variant To Data(error in=w308, Variant=w309) -> (error out=w307:errorcluster)  [unwired: 1 in, 1 out]
                  }
                  frame Enabled {
                  }
                }
                n93 = Bundle By Name(cluster=w302, "vData"=variant) -> (w301:T10)
              }
            }
            n94 = call <vilib>:"Add State(s) to Queue__JKI_lib_State_Machine.vi"("State(s) in Front (\"\")"=w285, "State(s) in (\"\")"=w293) -> ("States Out"=w292:string)  [unwired: 13 in]
          }
          event User Event {
            n95 = event-data() -> ("CmdMsg"=w317:string, "vData"=w321:variant)  [unwired: 1 in, 1 out]
            n96 = Unbundle By Name(w312) -> ("Self Reference"=w313:refnum<class "Application.lvclass">, "SMQ"=w311:refnum<queue>)
            n97 = call "get async msg.vi"("error in (no error)"=w319, "Msg String in"=w317) -> ("error out"=w318:errorcluster, "AsyncMsg"=w316:T20)  [unwired: 8 in]
            n98 = case shown="\"Application.AppClassReference\"" w316 {
              tunnel: w321 -> [_ w339]
              tunnel: w318 -> [w329 w338]
              tunnel: [w328 w333] -> w320
              tunnel: [_ ""] -> w315
              tunnel: w312 -> [w324 w336]
              tunnel: [w324 w335] -> w314
              tunnel: w313 -> [_ _]
              tunnel: w312 -> [_ _]
              tunnel: w311 -> [_ w332]
              frame Default {
                n99 = call <vilib>:"Build Error Cluster_ModKT .vi"("Prepend String (\"\")"="Invalid Async Cmd" ("Prepend String (\"\")"), "code"=42, "error? (F)"=TRUE, "error in (no error)"=w329) -> ("error out"=w328:errorcluster)  [unwired: 3 in, 1 out]
              }
              frame "Application.AppClassReference" {
                # "#NOTE: no need to update App class ref here,\nbut do update the status str control ref.\nReceiving this event implies Main UI is finished\ninitializing, including the status string."
                n100 = disable-structure shown="Disabled" {
                  disable-tunnel: w339 -> [w342 _]
                  disable-tunnel: w338 -> [w341 w343]
                  disable-tunnel: [w340 w343] -> w334
                  frame Disabled {
                    n101 = Variant To Data(error in=w341, Variant=w342) -> (error out=w340:errorcluster)  [unwired: 1 in, 1 out]
                  }
                  frame Enabled {
                  }
                }
                n102 = call <vilib>:"Add State to Queue with vData.vi"("queue in"=w332, "state in"="Action: UpdateSMData >> AppClassRef", "error in"=w334) -> ("error out"=w333:errorcluster)  [unwired: 9 in, 3 out]
                n103 = call "FG - StatusStrRef.vi"() -> ("StatusStr Ref out"=w330:refnum<vi>)  [unwired: 9 in, 1 out]
                n104 = Bundle By Name(cluster=w336, "StatusMsg Ref"=w330) -> (w335:T10)
              }
            }
            n105 = call <vilib>:"Add State(s) to Queue__JKI_lib_State_Machine.vi"("State(s) in Front (\"\")"=w315, "State(s) in (\"\")"=w323) -> ("States Out"=w322:string)  [unwired: 13 in]
          }
        }
      }
      frame "---------- Core ----------" {
        n106 = call <vilib>:"Add State(s) to Queue__JKI_lib_State_Machine.vi"("State(s) in (\"\")"=w349) -> ("States Out"=w348:string)  [unwired: 14 in]
      }
      frame "Initialize Core Data" {
        # "originally closed?"
        # "exe?"
        n107 = disable-structure shown="Enabled" {
          disable-tunnel: [w362 w366] -> w351
          frame Disabled {
            n108 = property class="App"() -> ("App.Kind"=w364:T15)  [unwired: 2 in, 2 out]
            n109 = Equal?(x=w364, y=T15."Run Time System" ("Application:Kind")) -> (x = y?=w362:bool)
          }
          frame Enabled {
            n110 = call "FG - FilePathnames.vi"("action (Get)"=TD_GetSet_ActionSelect--enum."Get") -> ("RunTimeSys?"=w366:bool)  [unwired: 3 in, 1 out]
          }
        }
        n111 = property class="VI"() -> ("Front Panel.Open"=w357:bool)  [unwired: 2 in, 2 out]
        n112 = control-ref of="Current VI Reference"() -> (w353:refnum<vi>)
        n113 = Not(x=w357) -> (.not. x?=w356:bool)
        n114 = Or(x=w356, y=w351) -> (x .or. y?=w354:bool)
        n115 = Bundle By Name(cluster=w355, "Core.Current VI Reference"=w353, "Core.Close Panel on Exit?"=w354, "RunTimeSystem?"=w351) -> (w359:T10)
        n116 = call <vilib>:"Add State(s) to Queue__JKI_lib_State_Machine.vi"("State(s) in (\"\")"=w361) -> ("States Out"=w360:string)  [unwired: 14 in]
      }
      frame "Process Sync" {
        n117 = Unbundle By Name(w372) -> ("process sync"=w371:refnum<notifier>)
        n118 = Send Notification(notification=TRUE, notifier=w371, error in (no error)=w369) -> (error out=w368:errorcluster)  [unwired: 1 out]
        n119 = call <vilib>:"Add State(s) to Queue__JKI_lib_State_Machine.vi"("State(s) in (\"\")"=w375) -> ("States Out"=w374:string)  [unwired: 14 in]
      }
      frame "DE_Register" {
        n120 = Unbundle By Name(w378) -> ("Public Events"=w377:T13)
        n121 = register-events(w377) -> (reference out=w380:refnum<event-registration>, error out=w379:errorcluster)  [unwired: 2 in]
      }
      frame "DE_Unregister" {
        n122 = Unregister For Events(event registration refnum=w384, error in=w383) -> ()  [unwired: 1 out]
      }
      frame "---------- Data ----------" {
        n123 = call <vilib>:"Add State(s) to Queue__JKI_lib_State_Machine.vi"("State(s) in (\"\")"=w392) -> ("States Out"=w391:string)  [unwired: 14 in]
      }
      frame "Data: InitializePostStartup" {
        n124 = Unbundle By Name(w394) -> ("SMQ"=w400:refnum<queue>)
        n125 = property class="Application.lvclass"(reference=w398) -> (reference out=w399:refnum<class "Application.lvclass">, "Accessors:Dependency*"=w393:T12)  [unwired: 1 in, 1 out]
        n126 = Bundle By Name(cluster=w394, "Dependency"=w393) -> (w395:T10)
        n127 = call <vilib>:"Add State to Queue with vData.vi"("queue in"=w400, "state in"="Action: UpdateSMData >> Dependency", "vData (\"\")"=w393, "error in"=w396) -> ("error out"=w397:errorcluster)  [unwired: 8 in, 3 out]
        n128 = call <vilib>:"Add State(s) to Queue__JKI_lib_State_Machine.vi"("State(s) in (\"\")"=w404) -> ("States Out"=w403:string)  [unwired: 14 in]
      }
      frame "Data: Initialize" {
        w409 = T21 {"Current VI Reference"=refnum, "Close Panel on Exit?"=FALSE}  # Core
        w411 = TRUE  # Your Boolean data
        w410 = ""  # Your string data
        # "process Self Reference is not live yet."
        n129 = disable-structure shown="Disabled" {
          disable-tunnel: w406 -> [w415 _]
          frame Disabled {
            n130 = Unbundle By Name(w415) -> ()  [unwired: 1 out]
          }
          frame Enabled {
          }
        }
        n131 = Bundle By Name(cluster=w406, "Core"=w409, "Your Boolean data"=w411, "Your string data"=w410) -> (w408:T10)
        n132 = call <vilib>:"Add State(s) to Queue__JKI_lib_State_Machine.vi"("State(s) in (\"\")"=w414) -> ("States Out"=w413:string)  [unwired: 14 in]
      }
      frame "Data: Cleanup" {
        n133 = Unbundle By Name(w418) -> ("Core.Current VI Reference"=w421:refnum<vi>)
        n134 = Close Reference(reference=w421, error in (no error)=w420) -> (error out=w419:errorcluster)
        n135 = call <vilib>:"Add State(s) to Queue__JKI_lib_State_Machine.vi"("State(s) in (\"\")"=w423) -> ("States Out"=w422:string)  [unwired: 14 in]
      }
      frame "---------- UI ----------" {
        n136 = call <vilib>:"Add State(s) to Queue__JKI_lib_State_Machine.vi"("State(s) in (\"\")"=w429) -> ("States Out"=w428:string)  [unwired: 14 in]
      }
      frame "UI: Initialize" {
        n137 = Unbundle By Name(w433) -> ("Core.Current VI Reference"=w432:refnum<vi>)
        n138 = call <userlib>:"Fit VI window to Largest Dec__ogtk.vi"("error in (no error)"=w435, "VI Ref (calling VI)"=w432) -> ("error out"=w434:errorcluster, "dup VI Ref"=w431:refnum<vi>)  [unwired: 4 in]
        n139 = disable-structure shown="Disabled" {
          disable-tunnel: w431 -> [w440 _]
          frame Disabled {
            n140 = property class="VI"(reference=w440, "Front Panel.Title"="*VI Title*" ("Front Panel Window:Title")) -> ()  [unwired: 1 in, 2 out]
          }
          frame Enabled {
          }
        }
        n141 = call <vilib>:"Add State(s) to Queue__JKI_lib_State_Machine.vi"("State(s) in (\"\")"=w438) -> ("States Out"=w437:string)  [unwired: 14 in]
      }
      frame "UI: Cursor Set" {
        # "Argument"
        n142 = case shown="\"Idle\", Default" w443 {
          tunnel: w445 -> [w450 w452]
          tunnel: [w449 w451] -> w444
          frame "Idle", Default {
            n143 = call <vilib>:"Unset Busy.vi"("error in (no error)"=w450) -> ("error out"=w449:errorcluster)  [unwired: 10 in]
          }
          frame "Busy" {
            n144 = call <vilib>:"Set Busy.vi"("error in (no error)"=w452) -> ("error out"=w451:errorcluster)  [unwired: 9 in, 1 out]
          }
        }
        n145 = call <vilib>:"Add State(s) to Queue__JKI_lib_State_Machine.vi"("State(s) in (\"\")"=w448) -> ("States Out"=w447:string)  [unwired: 14 in]
      }
      frame "UI: Front Panel State" {
        # "Argument"
        n146 = Unbundle By Name(w457) -> ("Core.Current VI Reference"=w456:refnum<vi>)
        n147 = case shown="\"Close\"" w455 {
          tunnel: w459 -> [w465 w478]
          tunnel: [w467 w479] -> w458
          tunnel: w456 -> [w466 w476]
          frame "Open", Default {
            n148 = property class="VI"(reference=w466, error in=w465) -> (reference out=w463:refnum<vi>, error out=w464:errorcluster, "Front Panel.Open"=w462:bool)
            n149 = case shown="False" w462 {
              tunnel: [w470 w473] -> w467
              tunnel: w464 -> [w469 w473]
              tunnel: w463 -> [w468 _]
              frame False {
                n150 = invoke class="VI" method="FP.Open"(reference=w468, error in=w469, "Activate"=TRUE, "State"=T17."Standard") -> (error out=w470:errorcluster)  [unwired: 1 in, 4 out]
              }
              frame True {
              }
            }
          }
          frame "Close" {
            n151 = property class="VI"(reference=w476, error in=w478) -> (reference out=w475:refnum<vi>, error out=w477:errorcluster, "Front Panel.Open"=w474:bool)
            n152 = case shown="True" w474 {
              tunnel: [w480 w483] -> w479
              tunnel: w477 -> [w480 w482]
              tunnel: w475 -> [_ w481]
              frame False {
              }
              frame True {
                n153 = invoke class="VI" method="FP.Close"(reference=w481, error in=w482) -> (error out=w483:errorcluster)  [unwired: 1 in, 2 out]
              }
            }
          }
        }
        n154 = call <vilib>:"Add State(s) to Queue__JKI_lib_State_Machine.vi"("State(s) in (\"\")"=w461) -> ("States Out"=w460:string)  [unwired: 14 in]
      }
      frame "---------- Macro ----------" {
        n155 = call <vilib>:"Add State(s) to Queue__JKI_lib_State_Machine.vi"("State(s) in (\"\")"=w489) -> ("States Out"=w488:string)  [unwired: 14 in]
      }
      frame "Macro: Initialize" {
        n156 = call <vilib>:"Add State(s) to Queue__JKI_lib_State_Machine.vi"("State(s) in Front (\"\")"=w491, "State(s) in (\"\")"=w496) -> ("States Out"=w495:string)  [unwired: 13 in]
      }
      frame "Macro: Exit" {
        n157 = Unbundle By Name(w505) -> ("Core.Close Panel on Exit?"=w504:bool)
        n158 = Select(t="UI: Front Panel State >> Close", s=w504, f="") -> (s? t:f=w501:string)
        n159 = call <vilib>:"Add State(s) to Queue__JKI_lib_State_Machine.vi"("State(s) in (\"\")"=w501, "State(s) at Back (\"\")"=w498) -> ("States Out"=w500:string)  [unwired: 13 in]
        n160 = call <vilib>:"Add State(s) to Queue__JKI_lib_State_Machine.vi"("State(s) in Front (\"\")"=w500, "State(s) in (\"\")"=w508) -> ("States Out"=w507:string)  [unwired: 13 in]
      }
      frame "---------- System ----------" {
        n161 = call <vilib>:"Add State(s) to Queue__JKI_lib_State_Machine.vi"("State(s) in (\"\")"=w514) -> ("States Out"=w513:string)  [unwired: 14 in]
      }
      frame "System: DisplayLaunchWindow" {
        # "splash screen header title string control label"
        n162 = Unbundle By Name(w530) -> ("Splash VI Ref"=w534:refnum<vi>, "Splash StatusRef"=w531:refnum<vi>, "StatusMsg Ref"=w532:refnum<vi>)
        n163 = property class="Str"(reference=w532) -> (error out=w516:errorcluster, "Value"=w520:string)  [unwired: 1 in, 1 out]
        n164 = call "FG - StatusStrRef.vi"("StatusStr Ref in"=w531, "error in (no error)"=w516, "action (Get)"=TD_GetSet_ActionSelect--enum."Set") -> ("StatusStr Ref out"=w518:refnum<vi>, "error out"=w517:errorcluster)  [unwired: 6 in]
        n165 = call <userlib>:"Set Control Value {Variant}__ogtk.vi"("error in (no error)"=w529, "Control Name (\"\": use variant name)"="FP Msg", "Value"="Quitting  IHS\nPlease Wait . . ." ("FP Msg"), "VI Refnum"=w534) -> ("error out"=w524:errorcluster, "VI Refnum dup"=w526:refnum<vi>)  [unwired: 6 in]
        n166 = property class="Str"(reference=w518, error in=w517, "Value"=w520) -> (reference out=w521:refnum<vi>, error out=w522:errorcluster)
        n167 = property class="VI"(reference=w526, error in=w524, "FP.Behavior"=T18."Modal" ("Front Panel Window:Behavior"), "FP.State"=T17."Standard" ("Front Panel Window:State")) -> (error out=w515:errorcluster)  [unwired: 1 out]
        n168 = property class="Str"(reference=w521, error in=w522, "Text.Scroll Position"=u32 999999999) -> ()  [unwired: 2 out]
        n169 = call <vilib>:"Add State(s) to Queue__JKI_lib_State_Machine.vi"("State(s) in (\"\")"=w538) -> ("States Out"=w537:string)  [unwired: 14 in]
      }
      frame "System: System Startup" {
        n170 = call "FG - StatusStrRef.vi"() -> ("StatusStr Ref out"=w543:refnum<vi>)  [unwired: 9 in, 1 out]
        n171 = call "System Startup.vi"("error in (no error)"=w546, "StatusStr ref"=w543, "Application in"=refnum<class "Application.lvclass"> refnum) -> ("error out"=w547:errorcluster, "Application out"=w545:refnum<class "Application.lvclass">)  [unwired: 7 in]
        n172 = case shown="Error" w547 {
          selector: w547 -> [_ w562]
          tunnel: ["" "Macro: Exit"] -> w544
          frame No Error {
          }
          frame Error {
            w558 = "\r\n"
            w564 = ""
            n173 = Unbundle(w562) -> ("source"=w559:string)  [unwired: 2 out]
            n174 = Concatenate Strings("System Startup Error.\nApplication cannot continue." ("message"), w558, w558, "===  Error Source ===", w558, w559, w558, "===============") -> (w556:string)
            n175 = call <vilib>:"Three Button Dialog.vi"("Window Title (\"\")"="SYSTEM ERROR" ("Window Title (\"\")"), "Right Button Text (\"Cancel\")"=w564, "Center Button Text (\"No\")"="OK" ("Left Button Text (\"Yes\")"), "Left Button Text (\"Yes\")"=w564, "message"=w556) -> ()  [unwired: 6 in, 1 out]
          }
        }
        n176 = property class="Application.lvclass"(reference=w545) -> (reference out=w542:refnum<class "Application.lvclass">, "Accessors:PublicEvents*"=w541:T13, "Accessors:Settings*"=w539:T11, "Accessors:Dependency*"=w540:T12)  [unwired: 1 in, 1 out]
        n177 = Bundle By Name(cluster=w548, "StatusMsg Ref"=w543, "Self Reference"=w542, "Public Events"=w541, "Settings"=w539, "Dependency"=w540) -> (w549:T10)
        n178 = call <vilib>:"Add State(s) to Queue__JKI_lib_State_Machine.vi"("State(s) in Front (\"\")"=w544, "State(s) in (\"\")"=w553) -> ("States Out"=w552:string)  [unwired: 13 in]
      }
      frame "System: Launch MainUI" {
        n179 = call "FG - FilePathnames.vi"() -> ("FilePaths out"=w575:T22)  [unwired: 4 in, 1 out]
        n180 = disable-structure shown="Disabled" {
          frame Disabled {
            n181 = vi-ref "ControlUI_Main.vi"() -> (w586:refnum<vi>)
            n182 = property class="VI" props=["Path"](reference=w586) -> ()  [unwired: 1 in, 3 out]
          }
          frame Enabled {
          }
        }
        n183 = Unbundle By Name(w575) -> ("MainUIPathname"=w566:path)
        n184 = Unbundle By Name(w571) -> ("Splash StatusRef"=w581:refnum<vi>, "Splash VI Ref"=w582:refnum<vi>, "Dependency.Main"=w570:refnum<class "Main.lvclass">)
        n185 = Open VI Reference(type specifier VI Refnum (for type only)=refnum<vi> refnum, vi path=w566, options=128, error in (no error)=w569) -> (vi reference=w574:refnum<vi>, error out=w576:errorcluster)  [unwired: 2 in]
        n186 = call-by-ref "Start Asynchronous Call"(reference=w574, error in=w576, "Splash StatusRef"=w581, "Splash VI Ref"=w582, "Application"=w567, "Main.lvclass"=w570) -> (reference out=w573:refnum<vi>, error out=w577:errorcluster)  [unwired: 8 in]
        n187 = call "FG - StatusStrRef.vi"() -> ("StatusStr Ref out"=w579:refnum<vi>)  [unwired: 9 in, 1 out]
        n188 = call <vilib>:"format status message v2.vi"("error in (no error)"=w569, "status msg"="Launching Main UI", "Str Refnum"=w579) -> ()  [unwired: 4 in, 5 out]
        n189 = Close Reference(reference=w573, error in (no error)=w577) -> (error out=w578:errorcluster)
        n190 = call <userlib>:"Clear All Errors__ogtk.vi"("Error In"=w578) -> ()  [unwired: 3 in, 1 out]
        n191 = call <vilib>:"Add State(s) to Queue__JKI_lib_State_Machine.vi"("State(s) in (\"\")"=w585) -> ("States Out"=w584:string)  [unwired: 14 in]
      }
      frame "System: ReturnLaunchState_Started" {
        n192 = case shown="\"Started\"" w589 {
          tunnel: [_ TD_LaunchState--enum."Started" ("LaunchState") TD_LaunchState--enum."Stopped" ("LaunchState")] -> w599
          frame Default {
          }
          frame "Started" {
          }
          frame "Stopped" {
          }
        }
        n193 = Unbundle By Name(w591) -> ("SMQ"=w594:refnum<queue>)
        n194 = Unbundle By Name(w591) -> ("LaunchState Ev"=w597:refnum<user-event>)
        n195 = Bundle By Name(cluster=T2 {"Time Stamp"=timestamp(0 s since 1904-01-01), "LaunchState"=enum."Started", "Error"={"status"=FALSE, "code"=0, "source"=""}} ("LaunchData"), "LaunchState"=w599) -> (w598:T2)
        n196 = Generate User Event(user event=w597, event data cluster=w598) -> (error out=w595:errorcluster)  [unwired: 2 in, 1 out]
        n197 = flat-sequence {
          tunnel: w591 -> [w606]
          tunnel: [w605] -> w593
          tunnel: w595 -> [_]
          tunnel: w587 -> [w604]
          tunnel: [w603] -> w588
          tunnel: w594 -> [w602]
          frame #0 {
            n198 = disable-structure shown="Disabled" {
              disable-tunnel: w606 -> [w614 w616]
              disable-tunnel: [w613 w616] -> w605
              disable-tunnel: w604 -> [w609 w615]
              disable-tunnel: [w608 w615] -> w603
              disable-tunnel: w602 -> [w607 _]
              frame Disabled {
                n199 = Bundle By Name(cluster=w614, "Initialized?"=TRUE) -> (w613:T10)
                n200 = call <vilib>:"Add State to Queue with vData.vi"("queue in"=w607, "state in"="Action: UpdateSMData >> Initialized", "vData (\"\")"=TRUE, "error in"=w609) -> ("error out"=w608:errorcluster)  [unwired: 8 in, 3 out]
              }
              frame Enabled {
              }
            }
          }
        }
        n201 = call <vilib>:"Add State(s) to Queue__JKI_lib_State_Machine.vi"("State(s) in (\"\")"=w590) -> ("States Out"=w592:string)  [unwired: 14 in]
      }
      frame "System: System Shutdown" {
        n202 = call "System Shutdown.vi"("error in (no error)"=w619, "Application in"=w621) -> ("error out"=w620:errorcluster)  [unwired: 8 in, 1 out]
        n203 = call <vilib>:"Add State(s) to Queue__JKI_lib_State_Machine.vi"("State(s) in (\"\")"=w625) -> ("States Out"=w624:string)  [unwired: 14 in]
      }
      frame "---------- Action ----------" {
        n204 = call <vilib>:"Add State(s) to Queue__JKI_lib_State_Machine.vi"("State(s) in (\"\")"=w631) -> ("States Out"=w630:string)  [unwired: 14 in]
      }
      frame "Action: Wait" {
        n205 = Scan From String(format string="%d", input string=w633, error in=w635, default 1=u32 0) -> (error out=w639:errorcluster, output 1=w638:u32)  [unwired: 1 in, 2 out]
        n206 = call <userlib>:"Wait (ms)__ogtk.vi"("error in (no error)"=w639, "milliseconds to wait"=w638) -> ("error out"=w634:errorcluster)  [unwired: 8 in, 1 out]
        n207 = call <vilib>:"Add State(s) to Queue__JKI_lib_State_Machine.vi"("State(s) in (\"\")"=w643) -> ("States Out"=w642:string)  [unwired: 14 in]
      }
      frame "Action: Terminate AsyncLoop" {
        n208 = Unbundle By Name(w650) -> ("SMQ"=w649:refnum<queue>)
        n209 = Flush Queue(queue=w649) -> (queue out=w648:refnum<queue>)  [unwired: 1 in, 2 out]
        n210 = call <vilib>:"Add State to Queue with vData.vi"("queue in"=w648, "state in"="Macro: Exit", "error in"=w646) -> ("error out"=w645:errorcluster)  [unwired: 9 in, 3 out]
        n211 = call <vilib>:"Add State(s) to Queue__JKI_lib_State_Machine.vi"("State(s) in (\"\")"=w653) -> ("States Out"=w652:string)  [unwired: 14 in]
      }
    }
  }
  n212 = Merge Errors(w7, w6) -> (w2:errorcluster)
  n213 = flat-sequence {
    tunnel: w1 -> [w655]
    tunnel: w2 -> [_]
    frame #0 {
      n214 = Unbundle By Name(w655) -> ("LaunchState Ev"=w656:refnum<user-event>)
      n215 = Generate User Event(user event=w656, event data cluster=T2 {"Time Stamp"=timestamp(0 s since 1904-01-01), "LaunchState"=enum."Stopped", "Error"={"status"=FALSE, "code"=0, "source"=""}} ("LaunchData")) -> ()  [unwired: 2 in, 2 out]
    }
  }
